vi "Abort.vi"(8 "error in (no error)":errorcluster, 11 "Object ref in":T1) -> (0 "error out":errorcluster, 3 "Object ref out":T1)   [LabVIEW 2013, in "SLMControl.lvlib" / "SC-Main.lvclass"]
uses:
  SC-Main.lvclass
  Object-reference.ctl
  SC-Main.lvclass/SC-Main.ctl
  Application-status.ctl
  Deposition-actions.ctl
  Lasing-actions.ctl
  UI/Control-names.ctl
  Read UI.vi
  Read Status.vi
  UI/Set-control-enable-multiple.vi
  UI/Set-control-boolean.vi
  UI/SC-UI.lvclass
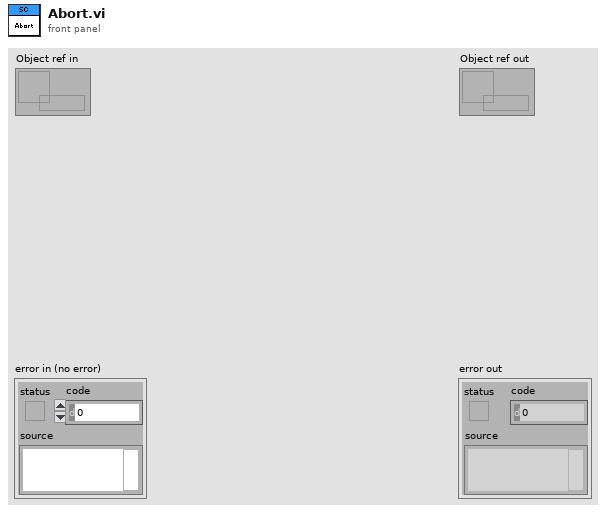
[diagram p1: front panel]
types:
  T1 = typedef "SLMControl.lvlib/SC-Main.lvclass/Object-reference.ctl" = refnum<data-value>
  T2 = typedef "SLMControl.lvlib/SC-UI.lvclass/Control-names.ctl" = enum16{"Com-in", "Com-out", "Help", "Status", "Load configuration", "Save configuration", "Load lasing files", "Load deposition files", "Clear", "Files", "Activate", "Execute", "Abort", "Options", "Current layer", "Current iteration", "Last elapsed time", "Deposition status", "Lasing job", "Status LEDs", "Exiting led", "Initialized led", "Files loaded led", "Activated led", "Executing led", "Deposition led", "Lasing job led", "Lasing led"}
  T3 = typedef "SLMControl.lvlib/SC-Main.lvclass/Lasing-actions.ctl" = enum16{"Idle", "Activate", "Load lasing file", "Launch lasing", "Wait for lasing end", "Signal iterate", "Signal abort", "Abort", "Reset", "Exit"}
  T4 = typedef "SLMControl.lvlib/SC-Main.lvclass/Deposition-actions.ctl" = enum16{"Idle", "Activate", "Load deposition", "Launch deposition", "Wait for deposition end", "Signal lasing", "Abort", "Reset", "Exit"}
  T5 = typedef "SLMControl.lvlib/SC-Main.lvclass/Application-status.ctl" = enum16{"Idle", "Initialized", "Configured", "Activated", "Started", "Paused", "Stopped", "Reset", "Error", "Exited"}
  T6 = typedef "SLMControl.lvlib/SC-Main.lvclass/Client-status.ctl" = enum16{"Idle", "Initialized", "Configured", "Activated", "Started", "Paused", "Stopped", "Reset", "Error", "Exited"}
  T7 = typedef "SLMControl.lvlib/SC-UI.lvclass/Panes-reference.ctl" = refnum<data-value>
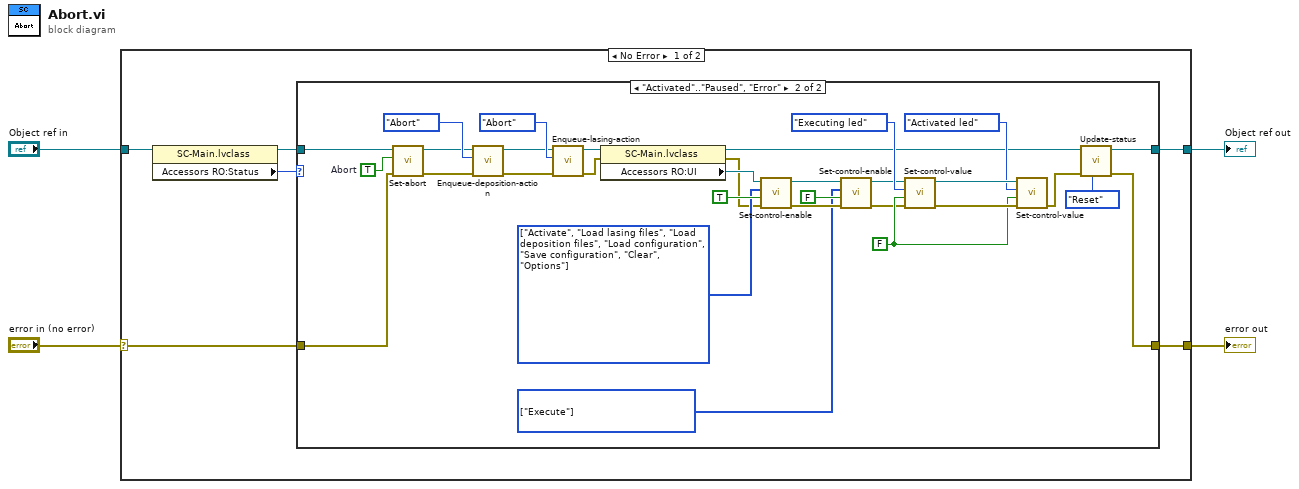
[diagram p0: block diagram]
diagram:
  n1 = case shown="No Error" "error in (no error)" {
    selector: "error in (no error)" -> [w10 w45]
    tunnel: [w9 w45] -> w3
    tunnel: [w8 w44] -> w1
    tunnel: "Object ref in" -> [w7 w44]
    frame No Error {
      n2 = property class="SC-Main.lvclass"(reference=w7) -> (reference out=w6:T1, "Accessors RO:Status"=w5:T6)  [unwired: 1 in, 1 out]
      n3 = case shown="\"Activated\"..\"Paused\", \"Error\"" w5 {
        tunnel: w6 -> [w12 w42]
        tunnel: w10 -> [w11 w41]
        tunnel: [w11 w39] -> w9
        tunnel: [w12 w38] -> w8
        frame Default {
        }
        frame "Activated".."Paused", "Error" {
          w18 = T2[] [enum."Execute"] items=["Com-in", "Com-out", "Help", "Status", "Load configuration", "Save configuration", "Load lasing files", "Load deposition files", "Clear", "Files", "Activate", "Execute", "Abort", "Options", "Current layer", "Current iteration", "Last elapsed time", "Deposition status", "Lasing job", "Status LEDs", "Exiting led", "Initialized led", "Files loaded led", "Activated led", "Executing led", "Deposition led", "Lasing job led", "Lasing led"] ("Control names")
          w21 = T2[] [enum."Activate", enum."Load lasing files", enum."Load deposition files", enum."Load configuration", enum."Save configuration", enum."Clear", enum."Options"] items=["Com-in", "Com-out", "Help", "Status", "Load configuration", "Save configuration", "Load lasing files", "Load deposition files", "Clear", "Files", "Activate", "Execute", "Abort", "Options", "Current layer", "Current iteration", "Last elapsed time", "Deposition status", "Lasing job", "Status LEDs", "Exiting led", "Initialized led", "Files loaded led", "Activated led", "Executing led", "Deposition led", "Lasing job led", "Lasing led"] ("Control names")
          w23 = FALSE
          w43 = TRUE  # Abort
          n4 = call "Set-abort.vi"("error in (no error)"=w41, "Abort"=w43, "Object ref in"=w42) -> ("error out"=w32:errorcluster, "Object ref out"=w33:T1)  [unwired: 7 in]
          n5 = call "Enqueue-deposition-action.vi"("error in (no error)"=w32, "Action"=Deposition-actions."Abort" ("Execution action"), "State queue in"=w33) -> ("error out"=w34:errorcluster, "State queue out"=w35:T1)  [unwired: 6 in, 1 out]
          n6 = call "Enqueue-lasing-action.vi"("error in (no error)"=w34, "Action"=Lasing-actions."Abort" ("Execution action"), "State queue in"=w35) -> ("error out"=w26:errorcluster, "State queue out"=w31:T1)  [unwired: 6 in, 1 out]
          n7 = property class="SC-Main.lvclass"(reference=w31, error in=w26) -> (reference out=w27:T1, error out=w13:errorcluster, "Accessors RO:UI"=w17:T7)
          n8 = call-poly "Set-control-enable.vi"("error in (no error)"=w13, "Enable?"=TRUE, "Control names"=w21, "Panes in"=w17) -> ("error out"=w20:errorcluster, "Panes out"=w16:T7)  [unwired: 6 in]
          n9 = call-poly "Set-control-enable.vi"("error in (no error)"=w20, "Enable?"=FALSE, "Control names"=w18, "Panes in"=w16) -> ("error out"=w14:errorcluster, "Panes out"=w15:T7)  [unwired: 6 in]
          n10 = call-poly "Set-control-value.vi"("error in (no error)"=w14, "Value"=w23, "Control name"=Control-names."Executing led", "Panes in"=w15) -> ("error out"=w25:errorcluster, "Panes out"=w30:T7)  [unwired: 6 in]
          n11 = call-poly "Set-control-value.vi"("error in (no error)"=w25, "Value"=w23, "Control name"=Control-names."Activated led", "Panes in"=w30) -> ("error out"=w24:errorcluster)  [unwired: 6 in, 1 out]
          n12 = call "Update-status.vi"("Status"=Application-status."Reset", "error in (no error)"=w24, "Object ref in"=w27) -> ("error out"=w39:errorcluster, "Object ref out"=w38:T1)  [unwired: 7 in]
        }
      }
    }
    frame Error {
    }
  }
  "error out" <- w3
  "Object ref out" <- w1
